vi "testEXT Data Identical Arrays.vi"(8 "error in (no error)":errorcluster, 11 "TestCase in":refnum<class "1D Array Test Case.lvclass">) -> (0 "error out":errorcluster, 3 "TestCase out":refnum<class "1D Array Test Case.lvclass">)   [LabVIEW 2015, in "1D Array Test Case.lvclass"]
uses:
  1D Array Test Case.lvclass
  <vilib>/addons/_JKI Toolkits/VI Tester/TestCase.llb/TestCase.lvclass
  VITAC.lvlib
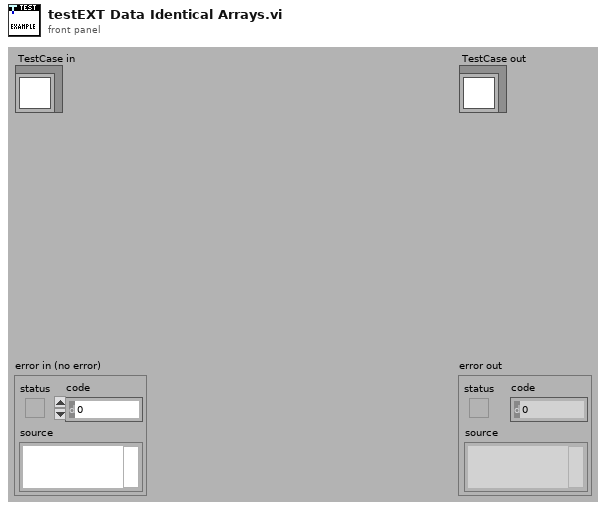
[diagram p1: front panel]
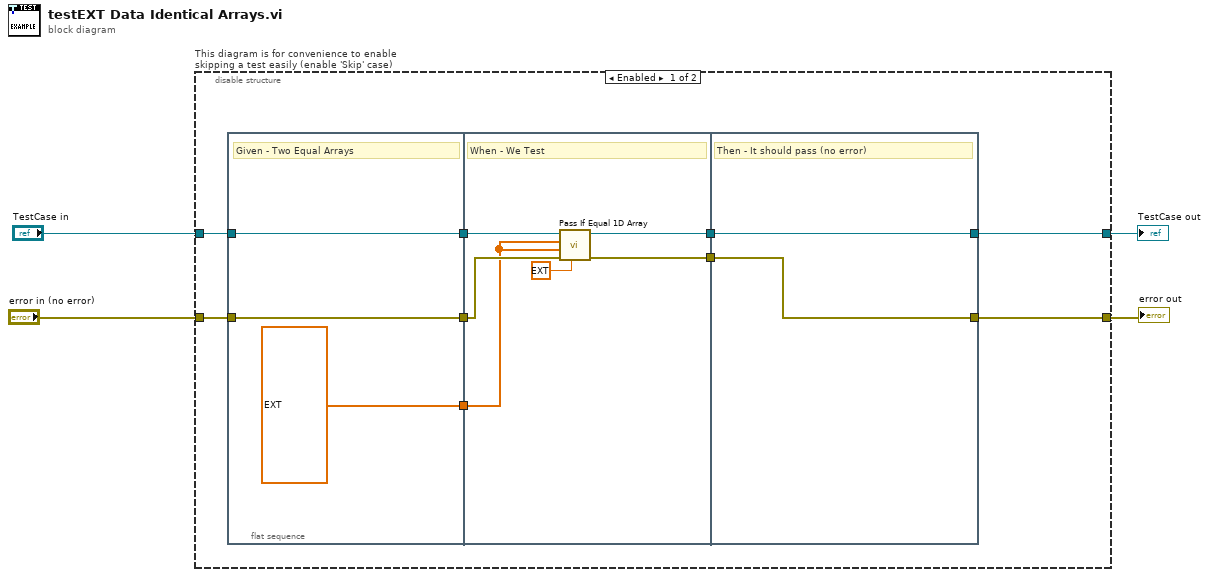
[diagram p0: block diagram]
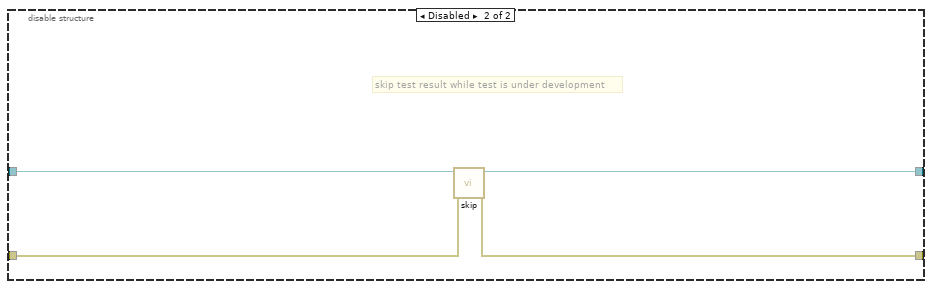
[diagram p2: hidden frame]
diagram:
  n1 = disable-structure "This diagram is for convenience to enable skipping a test easily (enable 'Skip' case)" shown="Enabled" {
    disable-tunnel: "TestCase in" -> [w12 w28]
    disable-tunnel: [w11 w26] -> w1
    disable-tunnel: [w7 w27] -> w3
    disable-tunnel: "error in (no error)" -> [w8 w25]
    frame Enabled {
      n2 = flat-sequence {
        tunnel: [w16] -> w13
        tunnel: w12 -> [w16]
        tunnel: [w15] -> w9
        tunnel: w8 -> [w15]
        tunnel: [ext[] [12.0, 13.0, 14.0, 15.0, 16.0, 17.0, 20000000000.0] ("x")] -> w5
        tunnel: w13 -> [w22]
        tunnel: [w21] -> w10
        tunnel: w9 -> [w20]
        tunnel: [w19] -> w6
        tunnel: w5 -> [w17]
        tunnel: [w24] -> w11
        tunnel: w10 -> [w24]
        tunnel: [w23] -> w7
        tunnel: w6 -> [w23]
        frame #0 {
          # "Given - Two Equal Arrays"
        }
        frame #1 {
          # "When - We Test"
          n3 = call "Pass If Equal 1D Array.vi"("delta (optional)"=ext 0.0, "error in (no error)"=w20, "actual"=w17, "expected"=w17, "TestCase in"=w22) -> ("error out"=w19:errorcluster, "TestCase out"=w21:refnum<class "1D Array Test Case.lvclass">)  [unwired: 5 in]
        }
        frame #2 {
          # "Then - It should pass (no error)"
        }
      }
    }
    frame Disabled {
      # "skip test result while test is under development"
      n4 = call <vilib>:"skip.vi"("error in (no error)"=w25, "TestCase in"=w28) -> ("error out"=w27:errorcluster, "TestCase out"=w26:refnum<class "1D Array Test Case.lvclass">)  [unwired: 8 in]
    }
  }
  "error out" <- w3
  "TestCase out" <- w1
